vi "Area.vi"(8 "error in (no error)":errorcluster, 11 "Text in":refnum<class "Text.lvclass">) -> (0 "error out":errorcluster, 2 "rect":T1, 3 "Text out":refnum<class "Text.lvclass">)   [LabVIEW 2021, in "Picture2D.lvlib" / "Text.lvclass"]
uses:
  Text.lvclass
  C:/GitHub/Picture2D/src/Picture2D/Picture2D.lvclass
  Font/Font.lvclass/Font.ctl
  Font/GetFontName.vi
  Font/GetSize.vi
  Font/GetStrikeout.vi
  Font/GetItalic.vi
  Font/GetUnderline.vi
  Font/GetOutline.vi
  Font/GetShadow.vi
  Font/GetBold.vi
  Font/Font.lvclass
  Point/Point.lvclass
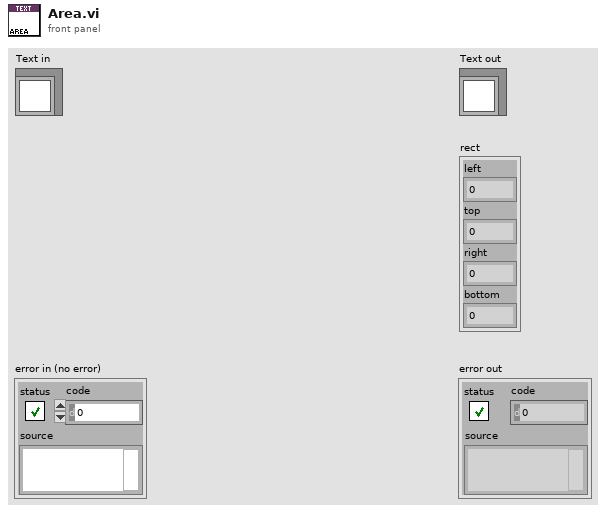
[diagram p1: front panel]
types:
  T1 = cluster{"left":i16, "top":i16, "right":i16, "bottom":i16}
  T2 = cluster{"Font Name:":string, "Size":i16, "Strikeout?":bool, "Italic?":bool, "Underline?":bool, "Outline?":bool, "Shadow?":bool, "Bold?":bool}
  T3 = enum16{"User-specified Font", "Application Font", "System Font", "Dialog Font"}
  T4 = cluster{"horizontal":enum16{"left", "center", "right"}, "vertical":enum16{"top", "center", "bottom"}}
  T5 = enum16{"None", "Stacked", "Clockwise", "Counterclockwise"}
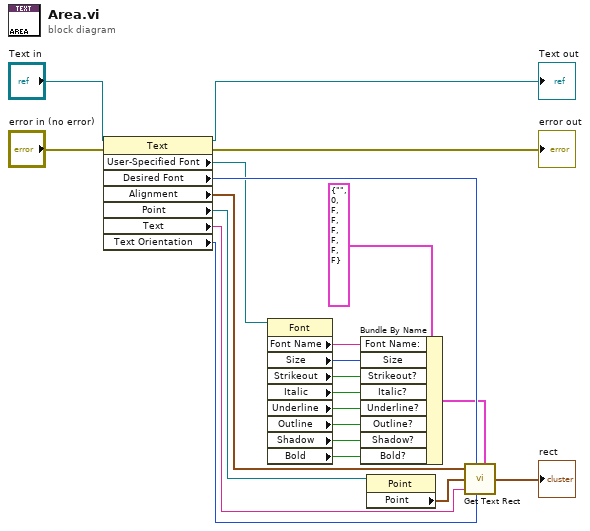
[diagram p0: block diagram]
diagram:
  n1 = property class="Text"(reference="Text in", error in="error in (no error)") -> (reference out=→"Text out":refnum<class "Text.lvclass">, error out=→"error out":errorcluster, "User-Specified Font"=w11:refnum<class "Font.lvclass">, "Desired Font"=w17:T3, "Alignment"=w20:T4, "Point"=w19:refnum<class "Point.lvclass">, "Text"=w15:string, "Text Orientation "=w14:T5)
  n2 = property class="Font"(reference=w11) -> ("Font Name"=w10:string, "Size"=w9:i16, "Strikeout"=w8:bool, "Italic"=w7:bool, "Underline"=w6:bool, "Outline"=w5:bool, "Shadow"=w4:bool, "Bold"=w3:bool)  [unwired: 1 in, 2 out]
  n3 = Bundle By Name(cluster=T2 {"Font Name:"="", "Size"=0, "Strikeout?"=FALSE, "Italic?"=FALSE, "Underline?"=FALSE, "Outline?"=FALSE, "Shadow?"=FALSE, "Bold?"=FALSE} ("[user-specified font]"), "Font Name:"=w10, "Size"=w9, "Strikeout?"=w8, "Italic?"=w7, "Underline?"=w6, "Outline?"=w5, "Shadow?"=w4, "Bold?"=w3) -> (w1:T2)
  n4 = property class="Point"(reference=w19) -> ("Point"=w18:cluster{"x":i16, "y":i16})  [unwired: 1 in, 2 out]
  n5 = call <vilib>:"Get Text Rect.vi"("alignment(left, top)"=w20, "desired font(Application)"=w17, "origin(0,0)"=w18, "text"=w15, "text orientation"=w14, "[user-specified font]"=w1) -> ("rect"=→"rect":T1)  [unwired: 3 in]
